vi "init_poller.vi"(8 "error in (no error)":errorcluster, 10 "input_poller in":refnum<class "input_poller.lvclass">, 11 "input in":refnum<class "input.lvclass">) -> (0 "error out":errorcluster, 3 "input out":refnum<class "input.lvclass">)   [LabVIEW 2015, in "input.lvclass"]
uses:
  input.lvclass
  input_poller/input_poller.lvclass
  input.lvclass/input.ctl
  input_poller/input_poller.lvclass/input_poller.ctl
  <vilib>/ActorFramework/Actor/Actor.lvclass
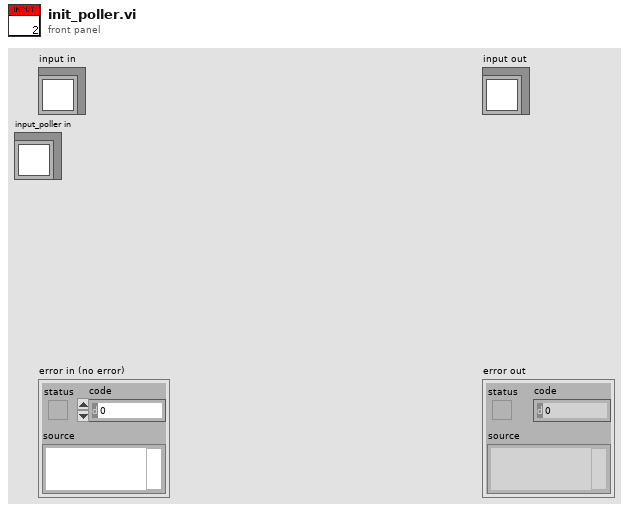
[diagram p1: front panel]
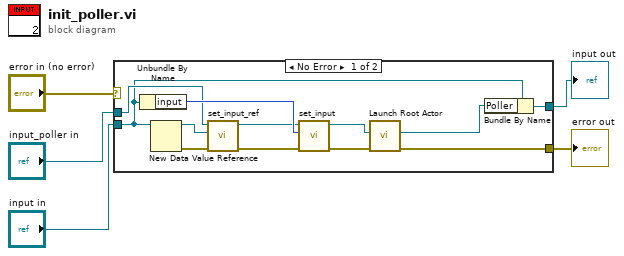
[diagram p0: block diagram]
diagram:
  n1 = case shown="No Error" "error in (no error)" {
    selector: "error in (no error)" -> [_ w19]
    tunnel: [w12 w19] -> w4
    tunnel: [w7 w18] -> w2
    tunnel: "input in" -> [w8 w18]
    tunnel: "input_poller in" -> [w9 _]
    frame No Error {
      n2 = Unbundle By Name(w8) -> ("input"=w17:i32)
      n3 = New Data Value Reference(data value=w8) -> (data value reference=w15:refnum<data-value>, error out=w16:errorcluster)  [unwired: 1 in]
      n4 = call "set_input_ref.vi"("error in (no error)"=w16, "input_ref"=w15, "input_poller in"=w9) -> ("error out"=w14:errorcluster, "input_poller out"=w13:refnum<class "input_poller.lvclass">)  [unwired: 7 in]
      n5 = call "set_input.vi"("error in (no error)"=w14, "input"=w17, "input_poller in"=w13) -> ("error out"=w11:errorcluster, "input_poller out"=w10:refnum<class "input_poller.lvclass">)  [unwired: 7 in]
      n6 = call <vilib>:"Launch Root Actor.vi"("error in (no error)"=w11, "Actor"=w10) -> ("error out"=w12:errorcluster, "Actor's Enqueuer"=w6:refnum<class "Message Enqueuer.lvclass">)  [unwired: 8 in]
      n7 = Bundle By Name(cluster=w8, "Poller"=w6) -> (w7:refnum<class "input.lvclass">)
    }
    frame Error {
    }
  }
  "error out" <- w4
  "input out" <- w2
